vi "Component Sweep Timing Test.vi"() -> ()   [LabVIEW 2015]
uses:
  Utility VIs/Math VIs/Math-Uniform Random Number (I32, scalar).vi
panel:
  out "Elapsed time (ms)":u32=70
  out "Phase Out":dbl[](array[numeric])
  in  "New Freq (Hz)":dbl=200.0
  in  "Last Freq (Hz)":dbl=100.0
  in  "Phase In":dbl
  out "Y":dbl[](array[numeric])=[0.9999999999901328, 0.9999999999901328, 0.9999999999901328, 0.9999999999901328, 0.9999999999901328, 0.9999999999901328, 0.9999999999901328, 0.9999999999901328, 0.9999999999901328, 0.9999999999901328, 0.9999999999901328, 0.9999999999901328, 0.9999999999901328, 0.9999999999901328, 0.9999999999901328, 0.9999999999901328, 0.9999999999901328, 0.9999999999901328, 0.9999999999901328, 0.9999999999901328, 0.9999999999901328, 0.9999999999901328, 0.9999999999901328, 0.9999999999901328, 0.9999999999901328, 0.9999999999901328, 0.9999999999901328, 0.9999999999901328, 0.9999999999901328, 0.9999999999901328, 0.9999999999901328, 0.9999999999901328, 0.9999999999901328, 0.9999999999901328, 0.9999999999901328, 0.9999999999901328, 0.9999999999901328, 0.9999999999901328, 0.9999999999901328, 0.9999999999901328, 0.9999999999901328, 0.9999999999901328, 0.9999999999901328, 0.9999999999901328, 0.9999999999901328, 0.9999999999901328, 0.9999999999901328, 0.9999999999901328, 0.9999999999901328, 0.9999999999901328, 0.9999999999901328, 0.9999999999901328, 0.9999999999901328, 0.9999999999901328, 0.9999999999901328, 0.9999999999901328, 0.9999999999901328, 0.9999999999901328, 0.9999999999901328, 0.9999999999901328, 0.9999999999901328, 0.9999999999901328, 0.9999999999901328, 0.9999999999901328, 0.9999999999901328, 0.9999999999901328, 0.9999999999901328, 0.9999999999901328, 0.9999999999901328, 0.9999999999901328, 0.9999999999901328, 0.9999999999901328, 0.9999999999901328, 0.9999999999901328, 0.9999999999901328, 0.9999999999901328, 0.9999999999901328, 0.9999999999901328, 0.9999999999901328, 0.9999999999901328, 0.9999999999901328, 0.9999999999901328, 0.9999999999901328, 0.9999999999901328, 0.9999999999901328, 0.9999999999901328, 0.9999999999901328, 0.9999999999901328, 0.9999999999901328, 0.9999999999901328, 0.9999999999901328, 0.9999999999901328, 0.9999999999901328, 0.9999999999901328, 0.9999999999901328, 0.9999999999901328, 0.9999999999901328, 0.9999999999901328, 0.9999999999901328, 0.9999999999901328]
  in  "Npts":i32=5000
  in  "dt (s)":dbl=0.02
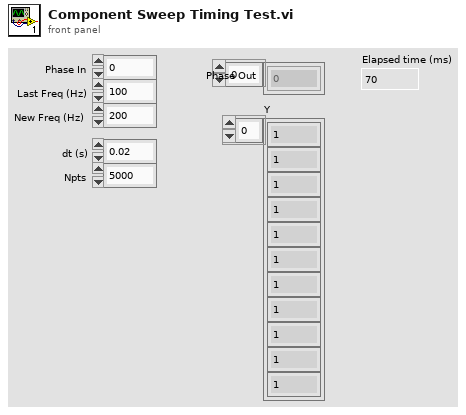
[diagram p1: front panel]
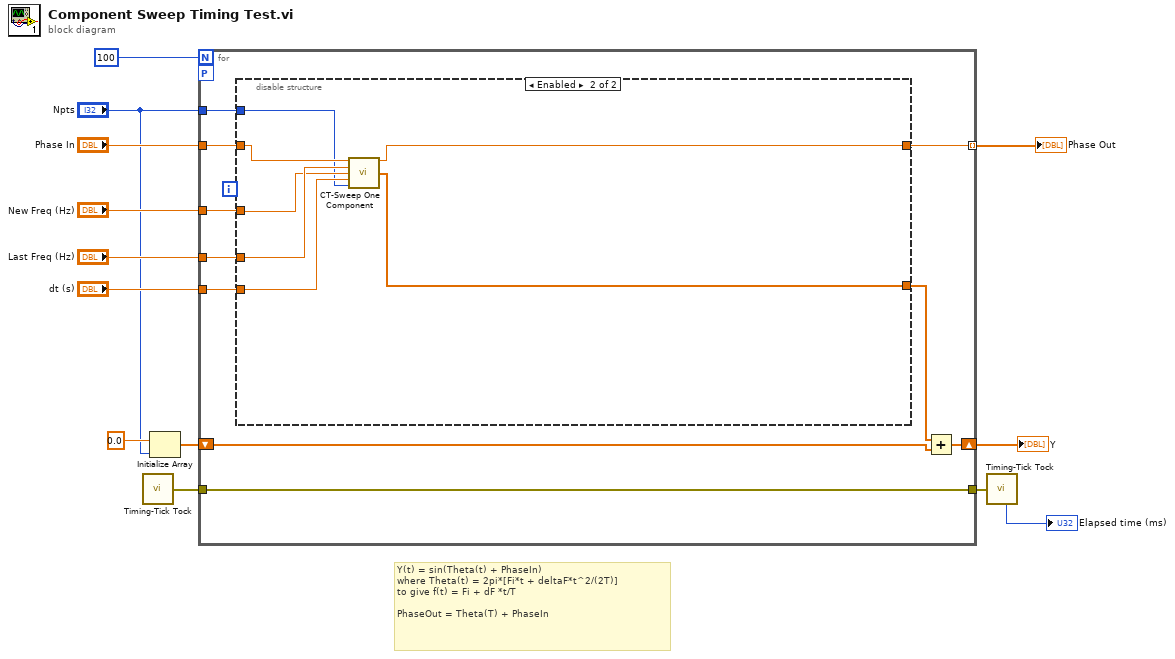
[diagram p0: block diagram]
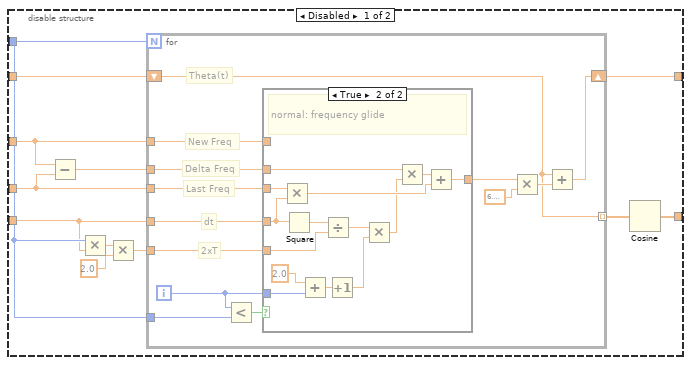
[diagram p2: hidden frame]
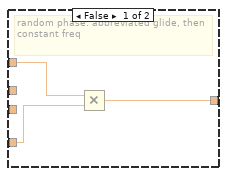
[diagram p3: hidden frame]
diagram:
  # "Y(t) = sin(Theta(t) + PhaseIn)\nwhere Theta(t) = 2pi*[Fi*t + deltaF*t^2/(2T)]\nto give f(t) = Fi + dF *t/T \n\nPhaseOut = Theta(T) + PhaseIn"
  n1 = call "Timing-Tick Tock.vi"() -> ("error out"=w9:errorcluster)  [unwired: 6 in, 1 out]
  n2 = Initialize Array(0.0 ("element"), "Npts") -> (w3:dbl[])
  n3 = for {
    N: 100 -> [_]
    tunnel: "Phase In" -> [w23]
    tunnel: "Last Freq (Hz)" -> [w22]
    tunnel: [w21] -> w11 mode=indexing
    tunnel: "dt (s)" -> [w18]
    tunnel: "Npts" -> [w19]
    tunnel: "New Freq (Hz)" -> [w20]
    shift-right: [w14] -> w2
    shift-left: w3 -> [w15]
    tunnel: w9 -> [w17]
    tunnel: [w17] -> w8
    workers-P: _ -> [_]
    n4 = disable-structure shown="Enabled" {
      disable-tunnel: w23 -> [w34 w72]
      disable-tunnel: w22 -> [w33 w71]
      disable-tunnel: [w32 w67] -> w21
      disable-tunnel: w20 -> [w29 w70]
      disable-tunnel: w19 -> [w28 w68]
      disable-tunnel: w18 -> [w27 w69]
      disable-tunnel: [w24 w66] -> w16
      frame Disabled {
        n5 = Subtract(x=w29, y=w33) -> (x-y=w30:dbl)
        n6 = Multiply(x=w28, y=w27) -> (x*y=w35:dbl)
        n7 = Multiply(x=w35, y=2.0) -> (x*y=w25:dbl)
        n8 = for {
          N: w28 -> [_]
          tunnel: w27 -> [w47]
          shift-right: [w43] -> w32
          shift-left: w34 -> [w42]
          tunnel: w33 -> [w48]
          tunnel: w25 -> [w40]
          tunnel: w30 -> [w41]
          tunnel: [w42] -> w26 mode=indexing
          tunnel: w28 -> [w37]
          tunnel: w29 -> [w36]
          i -> [w38]
          # "New Freq"
          # "dt"
          # "2xT"
          # "Theta(t)"
          # "Last Freq"
          # "Delta Freq"
          n9 = Less?(x=w38, y=w37) -> (x < y?=w39:bool)
          n10 = case shown="True" w39 {
            tunnel: w48 -> [_ w65]
            tunnel: w47 -> [w51 w64]
            tunnel: [w50 w59] -> w46
            tunnel: w41 -> [_ w58]
            tunnel: w40 -> [_ w57]
            tunnel: w38 -> [_ w55]
            tunnel: w36 -> [w49 _]
            frame False {
              # "random phase: abbreviated glide, then constant freq"
              n11 = Multiply(x=w49, y=w51) -> (x*y=w50:dbl)
            }
            frame True {
              # "normal: frequency glide"
              n12 = Multiply(x=w65, y=w64) -> (x*y=w60:dbl)
              n13 = Square(x=w64) -> (x^2=w63:dbl)
              n14 = Add(x=2.0, y=w55) -> (x+y=w53:dbl)
              n15 = Divide(x=w63, y=w57) -> (x/y=w62:dbl)
              n16 = Increment(x=w53) -> (x+1=w52:dbl)
              n17 = Multiply(x=w62, y=w52) -> (x*y=w56:dbl)
              n18 = Multiply(x=w58, y=w56) -> (x*y=w61:dbl)
              n19 = Add(x=w61, y=w60) -> (x+y=w59:dbl)
            }
          }
          n20 = Multiply(x=w46, y=6.283185307179586) -> (x*y=w44:dbl)
          n21 = Add(x=w42, y=w44) -> (x+y=w43:dbl)
        }
        n22 = Cosine(x=w26) -> (cos(x)=w24:dbl[])
      }
      frame Enabled {
        n23 = call "CT-Sweep One Component.vi"("Phase In"=w72, "Last Freq (Hz)"=w71, "New Freq (Hz)"=w70, "dt (s)"=w69, "Npts"=w68) -> ("Phase Out"=w67:dbl, "Y"=w66:dbl[])  [unwired: 9 in]
      }
    }
    n24 = Add(x=w16, y=w15) -> (x+y=w14:dbl[])
  }
  "Y" <- w2
  "Phase Out" <- w11
  n25 = call "Timing-Tick Tock.vi"("error in (no error)"=w8) -> ("Elapsed time (ms)"=→"Elapsed time (ms)":u32)  [unwired: 5 in, 1 out]
